vi "Get Status.vi"(8 "error in (no error)":errorcluster, 11 "Instrument.1820 in":refnum<class "Instrument.Oxford1820.lvclass">) -> (0 "error out":errorcluster, 1 "Status":T1, 2 "Status":string, 3 "Instrument.1820 in":refnum<class "Instrument.Oxford1820.lvclass">)   [LabVIEW 2019, in "Instrument.Oxford1820.lvclass"]
doc: "Status Bits:\n[0] = Hold?\n[1] = Ramp to Set?\n[2] = Ramp to Zero?\n[3] = Clamp?"
uses:
  Instrument.Oxford1820.lvclass
  Typedefs/Instrument.Oxford1820.protectedCommands-enum.ctl
  4a75fe41-9824-4f1c-9c0e-f041ee8b199c.vi/d5ceb21e-1b16-412d-b8ef-4d15fbf620d4.vi
  4a75fe41-9824-4f1c-9c0e-f041ee8b199c.vi/d5ceb21e-1b16-412d-b8ef-4d15fbf620d4.vi/89665312-4bb0-405b-847c-621473376f02.vi
  4a75fe41-9824-4f1c-9c0e-f041ee8b199c.vi/d5ceb21e-1b16-412d-b8ef-4d15fbf620d4.vi/b1efb1db-00fb-453b-9e78-4e5fec5d3ffc.vi
  <vilib>/Utility/Data Type/Get Type Information.vi
  <vilib>/JDP Science/JSONtext/JSON text to Variant.vi
  <vilib>/JDP Science/JSONtext/LVClass Serializer/JSONtext LVClass Serializer.lvclass
  98a4e1da-cb9d-4020-a1ae-9d5287634c87.vi
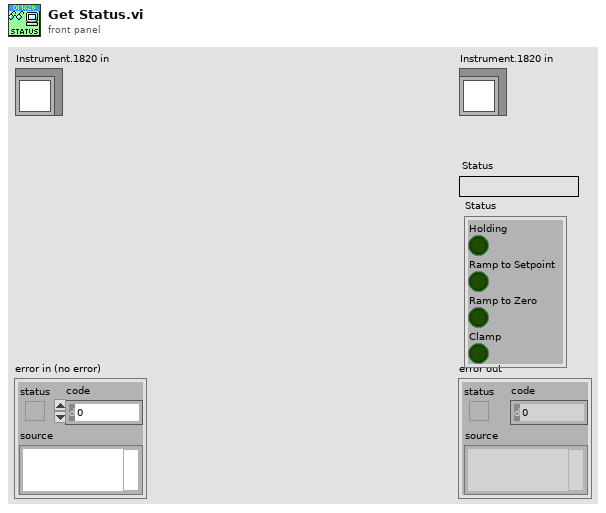
[diagram p1: front panel]
types:
  T1 = cluster{"Holding":bool, "Ramp to Setpoint":bool, "Ramp to Zero":bool, "Clamp":bool}
  T2 = typedef "Instrument.Oxford1820.lvclass/Instrument.Oxford1820.protectedCommands-enum.ctl" = enum16{"Hold", "RampToSet", "RampToZero", "Clamp", "setTarget", "setSwitchHeat", "setLambda", "setFillMode", "setNeedleValve", "getStatus", "getTarget", "getSwitchHeat", "getPSUField", "setSequenceStatus"}
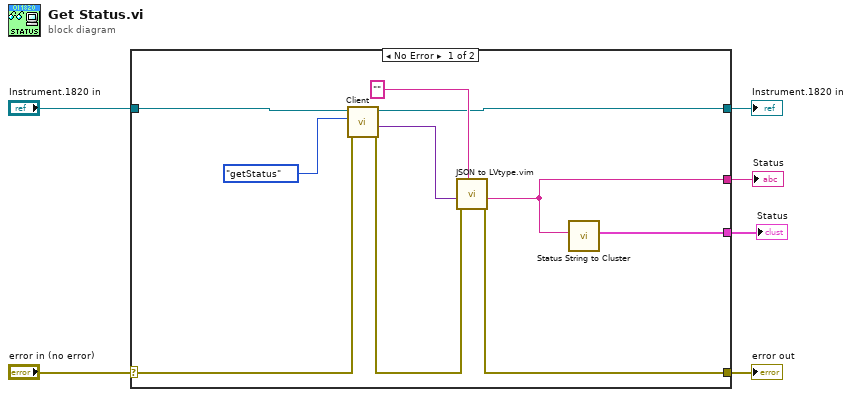
[diagram p0: block diagram]
diagram:
  n1 = case shown="No Error" "error in (no error)" {
    selector: "error in (no error)" -> [w14 w18]
    tunnel: [w12 w18] -> w5
    tunnel: [w10 w17] -> w3
    tunnel: "Instrument.1820 in" -> [w9 w17]
    tunnel: [w7 _] -> w2
    tunnel: [w16 _] -> w1
    frame No Error {
      n2 = call-dynamic "Client.vi"("error in (no error)"=w14, "Command in"=Instrument.Oxford1820.protectedCommands-enum."getStatus" ("Commands"), "Instrument in"=w9) -> ("error out"=w13:errorcluster, "Data out"=w15:variant, "Instrument out"=w10:refnum<class "Instrument.Oxford1820.lvclass">)  [unwired: 5 in, 1 out]
      n3 = call "JSON to LVtype.vim"("type"="", "error in (no error)"=w13, "JSON Data in"=w15) -> ("error out"=w12:errorcluster, "Data out"=w7:string)  [unwired: 7 in]
      n4 = call "Status String to Cluster.vi"("Status String"=w7) -> ("Status"=w16:T1)  [unwired: 10 in]
    }
    frame Error {
    }
  }
  "error out" <- w5
  "Instrument.1820 in" <- w3
  "Status" <- w2
  "Status" <- w1
